vi "Reset.vi"(7 "1-Wire DIO Pin":refnum<k21>="ConnectorA/DIO15", 8 "error in":errorcluster) -> (0 "error out":errorcluster, 1 "0 = Device Present / 1=no":bool)   [LabVIEW 2014, in "Maxim 1-Wire.lvlib"]
doc: "INITIALIZATION\nAll transactions on the 1-Wire bus begin with an initialization sequence. The initialization sequence consists of a reset pulse transmitted by the bus master followed by presence pulse(s) transmitted by the slave(s). The presence pulse lets the bus master know that slave devices (such as the DS18B20) are on the bus and are ready to operate. Timing for the reset and presence pulses is detailed in the 1-Wire Signaling section.\n\n\nThis VI is created by Vincent Claes for FPDA-1 more information on http://pwo.fpga.be\n\nvincent.claes@xios.be\nclaesvincent@gmail.com\n\nhttp://www.linkedin.com/in/vincentclaes"
uses:
  Maxim 1-Wire.lvlib
  <vilib>/rvi/Emulation/niFpgaSctlEmulationGetInTimedLoop.vi
  <vilib>/rvi/Emulation/niFpgaProcessEmulError.vi
  <vilib>/rvi/eio/common/nirviEmuTemplateMethod_errors.vi
  <vilib>/eio/EIOMethodNode/EIOMethodNode.xnode
  <vilib>/eio/EIONode/EIONode.xnode
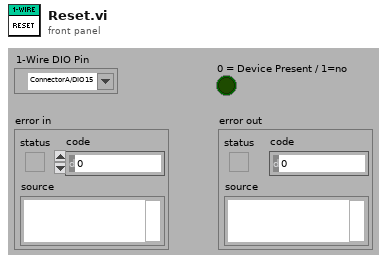
[diagram p1: front panel]
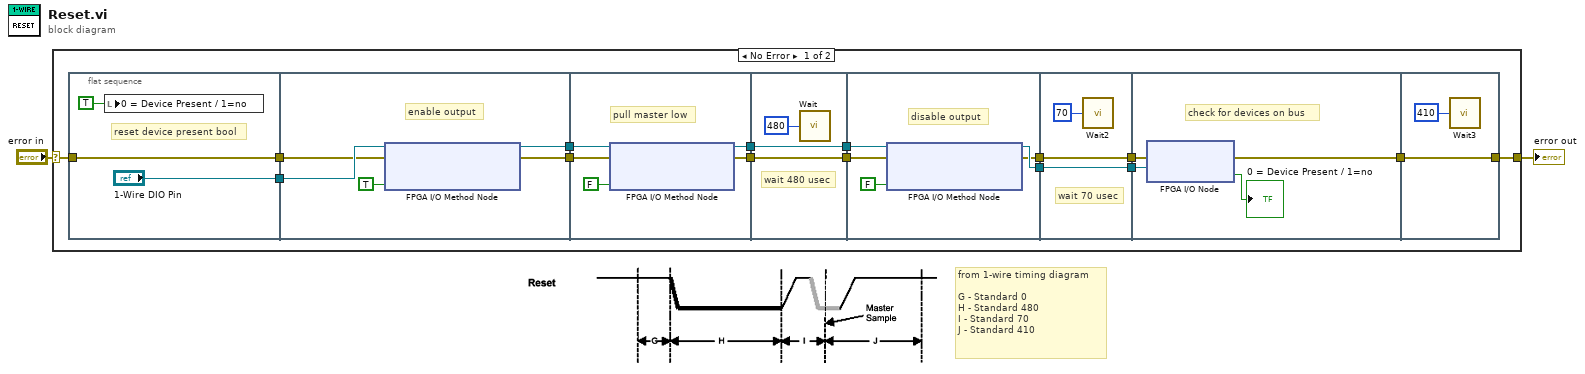
[diagram p0: block diagram]
diagram:
  # "from 1-wire timing diagram\n\nG - Standard 0\nH - Standard 480\nI - Standard 70\nJ - Standard 410"
  n1 = case shown="No Error" "error in" {
    selector: "error in" -> [w3 w48]
    tunnel: [w4 w48] -> w2
    frame No Error {
      n2 = flat-sequence {
        tunnel: ["1-Wire DIO Pin"] -> w17
        tunnel: [w18] -> w16
        tunnel: w3 -> [w18]
        tunnel: [w24] -> w15
        tunnel: [w23] -> w14
        tunnel: w17 -> [w22]
        tunnel: w16 -> [w21]
        tunnel: w15 -> [w30]
        tunnel: w14 -> [w29]
        tunnel: [w28] -> w13
        tunnel: [w27] -> w12
        tunnel: [w32] -> w11
        tunnel: w13 -> [w32]
        tunnel: w12 -> [w31]
        tunnel: [w31] -> w10
        tunnel: [w37] -> w9
        tunnel: [w36] -> w8
        tunnel: w11 -> [w35]
        tunnel: w10 -> [w34]
        tunnel: [w40] -> w7
        tunnel: w9 -> [w40]
        tunnel: w8 -> [w39]
        tunnel: [w39] -> w6
        tunnel: w7 -> [w44]
        tunnel: w6 -> [w43]
        tunnel: [w42] -> w5
        tunnel: w5 -> [w46]
        tunnel: [w46] -> w4
        frame #0 {
          # "reset device present bool"
          n3 = local write "0 = Device Present / 1=no"(TRUE ("0 = Device Present / 1=no")) -> ()
        }
        frame #1 {
          # "enable output"
          n4 = xnode "FPGA I/O Method Node"("error in"=w21, "FPGA I/O In"=w22, "Enable"=TRUE ("Data")) -> ("error out"=w23:errorcluster, "FPGA I/O Out"=w24:refnum<k21>)
        }
        frame #2 {
          # "pull master low"
          n5 = xnode "FPGA I/O Method Node"("error in"=w29, "FPGA I/O In"=w30, "Data"=FALSE ("FX2_IO1_J1_0")) -> ("error out"=w27:errorcluster, "FPGA I/O Out"=w28:refnum<k21>)
        }
        frame #3 {
          # "wait 480 usec"
          n6 = call "Wait"("Count(uSec)"=u32 480) -> ()  [unwired: 1 out]
        }
        frame #4 {
          # "disable output"
          n7 = xnode "FPGA I/O Method Node"("error in"=w34, "FPGA I/O In"=w35, "Enable"=FALSE ("Data")) -> ("error out"=w36:errorcluster, "FPGA I/O Out"=w37:refnum<k21>)
        }
        frame #5 {
          # "wait 70 usec"
          n8 = call "Wait2"("Count(uSec)"=u32 70) -> ()  [unwired: 1 out]
        }
        frame #6 {
          # "check for devices on bus"
          n9 = xnode "FPGA I/O Node"("error in"=w43, "FPGA I/O In"=w44) -> ("error out"=w42:errorcluster, "I/O Item"=→"0 = Device Present / 1=no":bool)  [unwired: 1 out]
        }
        frame #7 {
          n10 = call "Wait3"("Count(uSec)"=u32 410) -> ()  [unwired: 1 out]
        }
      }
    }
    frame Error {
    }
  }
  "error out" <- w2
